vi "Check Exposure.vi"(8 "error in (no error)":errorcluster, 11 "Scan Data Process in":T1) -> (0 "error out":errorcluster, 2 "Combine?":string, 3 "Scan Data Process out":T1)   [LabVIEW 2015, in "Exposure Process.lvlib"]
uses:
  Exposure Process.lvlib
  Control_Scan Data Process.ctl
  <vilib>/addons/PointValueMap/controls/PointMap.ctl
  Control_EXP Information.ctl
  Control_File Save Setup.ctl
  Control_Enable and Path.ctl
  Control_ICM Export Setting.ctl
  <vilib>/addons/PointValueMap/PointValueMap.lvlib
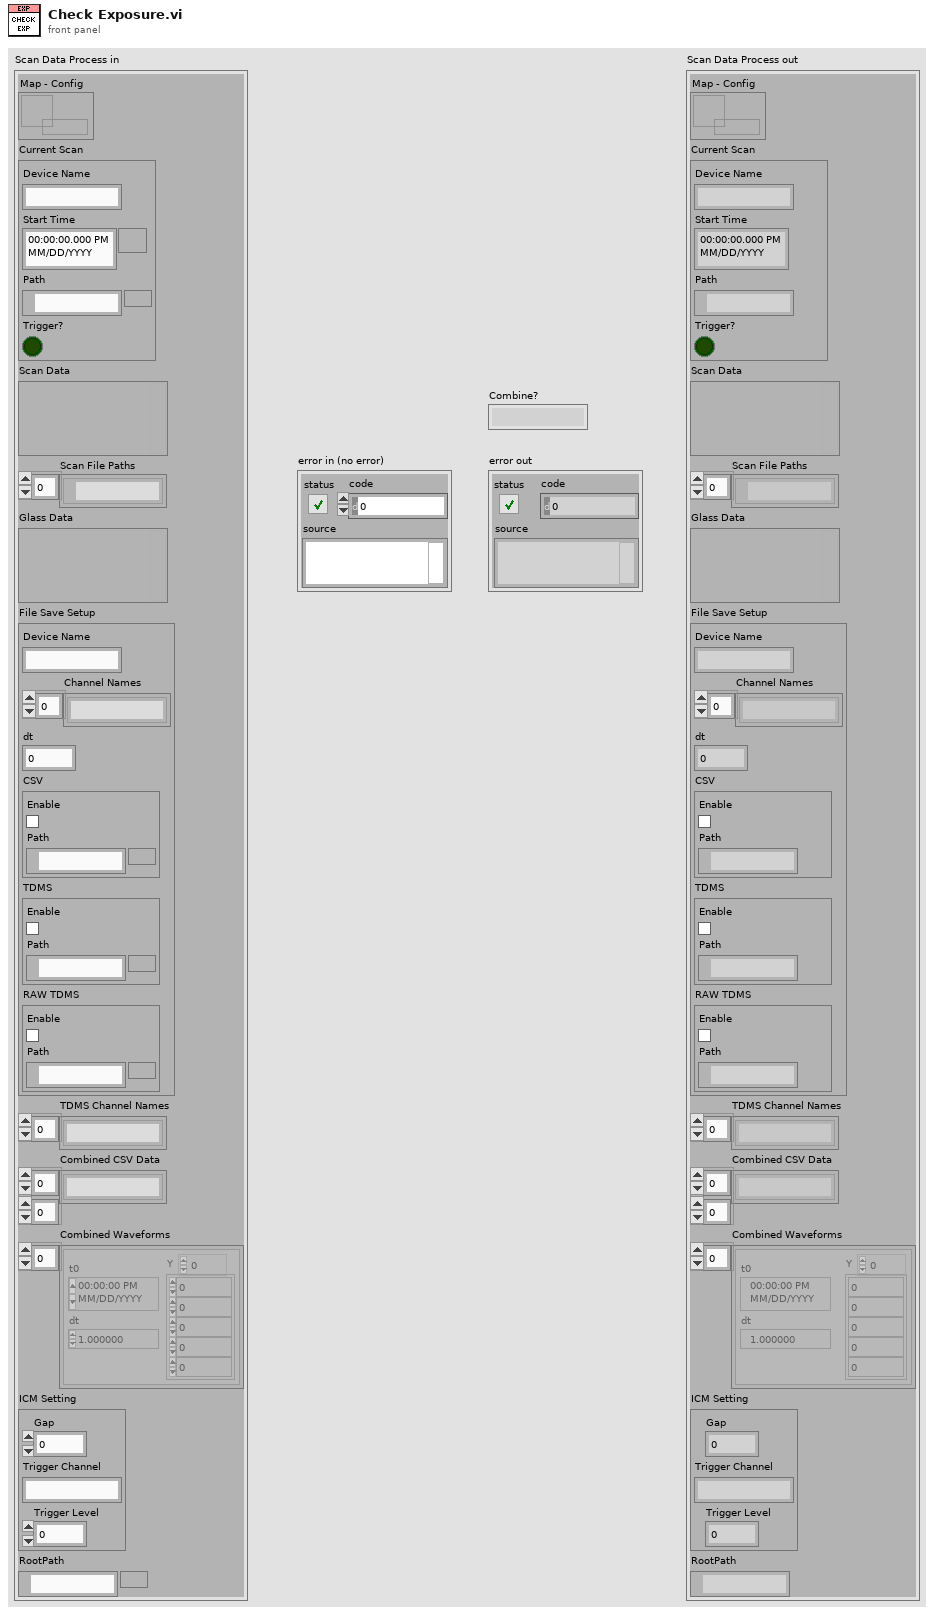
[diagram p1: front panel]
types:
  T1 = typedef "Exposure Process.lvlib/Control_Scan Data Process.ctl" = cluster{"Map - Config":T2, "Current Scan":T3, "Scan Data":variant, "Scan File Paths":path[], "Glass Data":variant, "File Save Setup":T4, "TDMS Channel Names":string[], "Combined CSV Data":string[][], "Combined Waveforms":waveform(dbl)[], "ICM Setting":T6, "RootPath":path}
  T2 = typedef "PointValueMap.lvlib/PointMap.ctl" = refnum<data-value>
  T3 = typedef "Exposure Process.lvlib/Control_EXP Information.ctl" = cluster{"Device Name":string, "Start Time":timestamp, "Path":path, "Trigger?":bool}
  T4 = typedef "Exposure Process.lvlib/Control_File Save Setup.ctl" = cluster{"Device Name":string, "Channel Names":string[], "dt":dbl, "CSV":T5, "TDMS":T5, "RAW TDMS":T5}
  T5 = typedef "Exposure Process.lvlib/Control_Enable and Path.ctl" = cluster{"Enable":bool, "Path":path}
  T6 = typedef "Exposure Process.lvlib/Control_ICM Export Setting.ctl" = cluster{"Gap":dbl, "Trigger Channel":string, "Trigger Level":dbl}
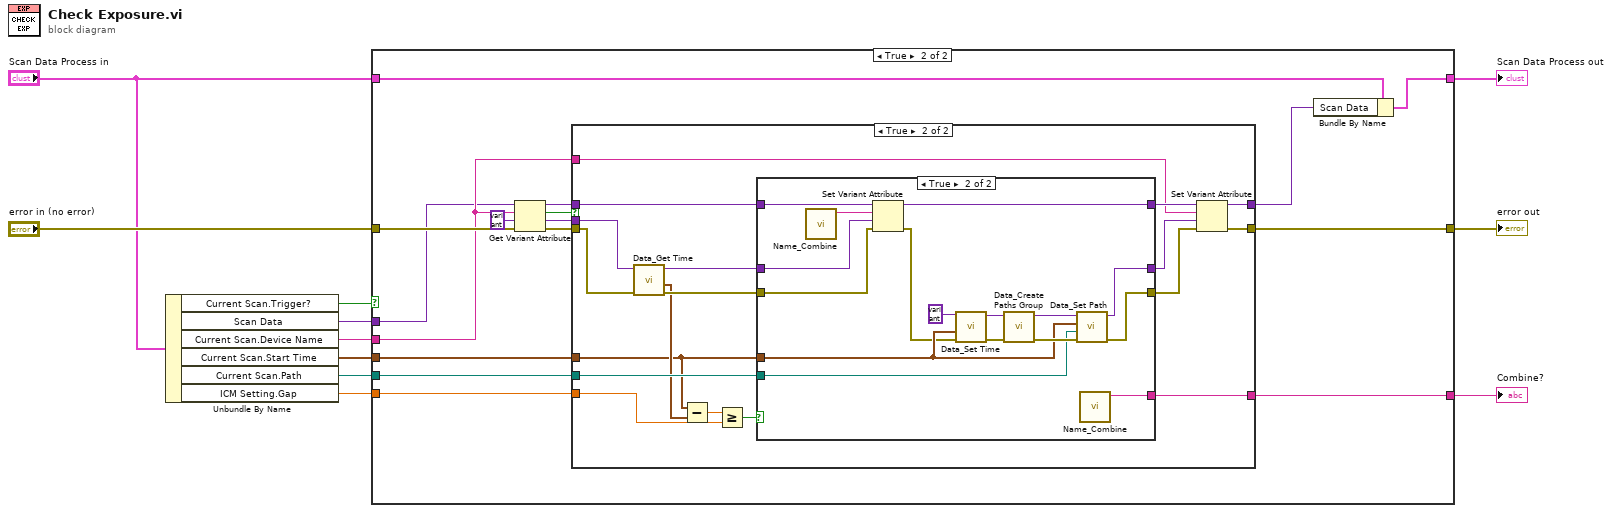
[diagram p0: block diagram]
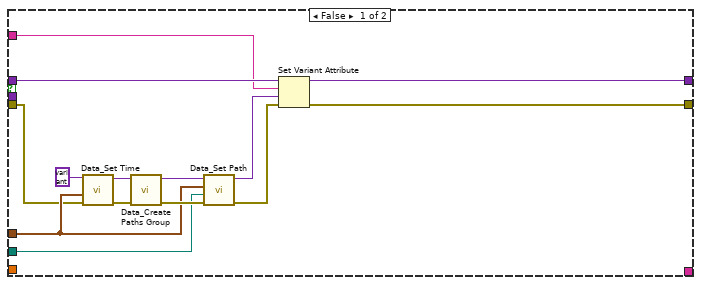
[diagram p3: hidden frame]
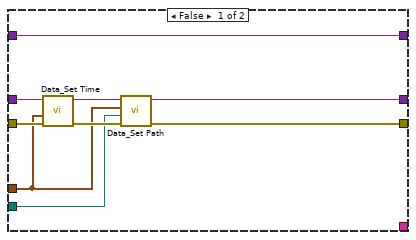
[diagram p4: hidden frame]
diagram:
  n1 = Unbundle By Name("Scan Data Process in") -> ("Current Scan.Trigger?"=w2:bool, "Scan Data"=w5:variant, "Current Scan.Device Name"=w6:string, "Current Scan.Start Time"=w7:timestamp, "Current Scan.Path"=w8:path, "ICM Setting.Gap"=w1:dbl)
  n2 = case shown="True" w2 {
    tunnel: "error in (no error)" -> [w12 w24]
    tunnel: [w12 w23] -> w10
    tunnel: [_ w22] -> w9
    tunnel: w8 -> [_ w21]
    tunnel: w7 -> [_ w20]
    tunnel: w6 -> [_ w19]
    tunnel: w5 -> [_ w18]
    tunnel: "Scan Data Process in" -> [w13 w16]
    tunnel: [w13 w15] -> w3
    tunnel: w1 -> [_ w14]
    frame False {
    }
    frame True {
      n3 = Get Variant Attribute(Variant=w18, name=w19, default value (empty Variant)=variant, error in=w24) -> (duplicate Variant=w28:variant, found=w29:bool, value=w26:variant, error out=w27:errorcluster)
      n4 = case shown="True" w29 {
        tunnel: w28 -> [w36 w55]
        tunnel: w20 -> [w37 w45]
        tunnel: w21 -> [w38 w58]
        tunnel: w19 -> [w34 w53]
        tunnel: w27 -> [w33 w60]
        tunnel: w26 -> [_ w61]
        tunnel: [w31 w50] -> w17
        tunnel: [w30 w49] -> w23
        tunnel: [_ w48] -> w22
        tunnel: w14 -> [_ w44]
        frame False {
          n5 = call "Data_Set Time.vi"("error in (no error)"=w33, "Time Stamp"=w37, "variant"=variant) -> ("error out"=w41:errorcluster, "variant out"=w42:variant)  [unwired: 7 in]
          n6 = call "Data_Create Paths Group.vi"("error in (no error)"=w41, "variant"=w42) -> ("error out"=w39:errorcluster, "variant out"=w40:variant)  [unwired: 8 in]
          n7 = call "Data_Set Path.vi"("error in (no error)"=w39, "Path"=w38, "Time Stamp"=w37, "variant"=w40) -> ("error out"=w32:errorcluster, "variant out"=w35:variant)  [unwired: 6 in]
          n8 = Set Variant Attribute(Variant=w36, name=w34, value=w35, error in=w32) -> (Variant out=w31:variant, error out=w30:errorcluster)  [unwired: 1 out]
        }
        frame True {
          n9 = call "Data_Get Time.vi"("error in (no error)"=w60, "variant"=w61) -> ("error out"=w56:errorcluster, "Last Start Time"=w46:timestamp, "variant out"=w57:variant)  [unwired: 7 in]
          n10 = Subtract(x=w45, y=w46) -> (x-y=w47:dbl)
          n11 = Greater Or Equal?(x=w47, y=w44) -> (x >= y?=w59:bool)
          n12 = case shown="True" w59 {
            tunnel: w45 -> [w66 w80]
            tunnel: w58 -> [w65 w81]
            tunnel: w57 -> [w70 w72]
            tunnel: w56 -> [w69 w71]
            tunnel: [w64 w78] -> w52
            tunnel: [w63 w79] -> w51
            tunnel: w55 -> [w62 w77]
            tunnel: [w62 w76] -> w54
            tunnel: [_ w73] -> w48
            frame False {
              n13 = call "Data_Set Time.vi"("error in (no error)"=w69, "Time Stamp"=w66, "variant"=w70) -> ("error out"=w67:errorcluster, "variant out"=w68:variant)  [unwired: 7 in]
              n14 = call "Data_Set Path.vi"("error in (no error)"=w67, "Path"=w65, "Time Stamp"=w66, "variant"=w68) -> ("error out"=w63:errorcluster, "variant out"=w64:variant)  [unwired: 6 in]
            }
            frame True {
              n15 = call "Name_Combine.vi"() -> ("Name"=w74:string)  [unwired: 11 in]
              n16 = Set Variant Attribute(Variant=w77, name=w74, value=w72, error in=w71) -> (Variant out=w76:variant, error out=w75:errorcluster)  [unwired: 1 out]
              n17 = call "Data_Set Time.vi"("error in (no error)"=w75, "Time Stamp"=w80, "variant"=variant) -> ("error out"=w84:errorcluster, "variant out"=w85:variant)  [unwired: 7 in]
              n18 = call "Data_Create Paths Group.vi"("error in (no error)"=w84, "variant"=w85) -> ("error out"=w82:errorcluster, "variant out"=w83:variant)  [unwired: 8 in]
              n19 = call "Data_Set Path.vi"("error in (no error)"=w82, "Path"=w81, "Time Stamp"=w80, "variant"=w83) -> ("error out"=w79:errorcluster, "variant out"=w78:variant)  [unwired: 6 in]
              n20 = call "Name_Combine.vi"() -> ("Name"=w73:string)  [unwired: 11 in]
            }
          }
          n21 = Set Variant Attribute(Variant=w54, name=w53, value=w52, error in=w51) -> (Variant out=w50:variant, error out=w49:errorcluster)  [unwired: 1 out]
        }
      }
      n22 = Bundle By Name(cluster=w16, "Scan Data"=w17) -> (w15:T1)
    }
  }
  "error out" <- w10
  "Combine?" <- w9
  "Scan Data Process out" <- w3
